vi "TeledyneMFC.vi"(7 "Value to Output":dbl format="%.2f", 8 "Ch Description":T1={"Ch Name"="TeleVue:Mdot:Meas(g/min)", "Type"="Run VI Named:", "Function"=enum."Analogue Output", "Ch State"=enum."On", "Calibration type"="Raw", "A"=0.0, "B"=0.0, "C"=0.0, "D"=0.0, "Comments"="!ASYNC", "Address"={"Main"=186, "Ch."=0, "Sub"=0, "Port Name"="tcp://192.168.124.71:10001"}, "String"="Front Panel", "Duty"=65535} {"Duty" format="%016b"; "D" format="%#_5g"; "C" format="%#_5g"; "B" format="%#_5g"; "A" format="%#_5g"}) -> (0 "Scan comment":string, 1 "Output":dbl=nan format="%.3f", 3 "HelpText":string="Analogue Input: Reads flowrate\nAnalogue Output: Sets digital control, sets setpoint, puts valve in auto\nNegative demand will ForceValveClosed\nDigital Output: 0-forceClosed, else-Automatic")   [LabVIEW 2017]
uses:
  ADAM Client/Sub VIs/ADAM Controls/Ch_description_ADAM.ctl
  ADAM Client/Sub VIs/ADAM Controls/Module_type_ADAM.ctl
  ADAM Client/Sub VIs/ADAM Controls/Function_ADAM.ctl
  ADAM Client/Sub VIs/ADAM Controls/Channel_State.ctl
  ADAM Client/Sub VIs/ADAM Controls/Calib_type_ADAM.ctl
  ADAM Client/Sub VIs/ADAM Controls/Address.ctl
  subVIs/TeledyneVueCommand.ctl
panel:
  out "GoodComms":bool
  # "VI to control Teledyne Vue Mass Flow Controller"
  # "http://www.teledyne-hi.com/products-services/thermal-mass-flow/300-vue-series"
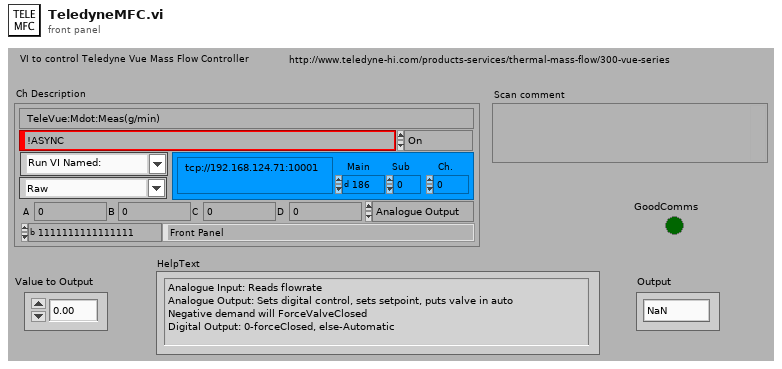
[diagram p1: front panel]
types:
  T1 = typedef "Ch_description_ADAM.ctl" = cluster{"Ch Name":string, "Type":T2, "Function":T3, "Ch State":T4, "Calibration type":T5, "A":dbl, "B":dbl, "C":dbl, "D":dbl, "Comments":string, "Address":T6, "String":string, "Duty":u16}
  T2 = typedef "Module_type_ADAM.ctl" = string
  T3 = typedef "Function_ADAM.ctl" = enum16{"Analogue Input", "Digital Input", "Event counter", "Event rate", "Analogue Output", "Digital Output", "Relay Output"}
  T4 = typedef "Channel_State.ctl" = enum16{"On", "Off", "Always On", "Always Off"}
  T5 = typedef "Calib_type_ADAM.ctl" = string
  T6 = typedef "Address.ctl" = cluster{"Main":i32, "Ch.":i32, "Sub":i32, "Port Name":string}
  T7 = typedef "TeledyneVueCommand.ctl" = string
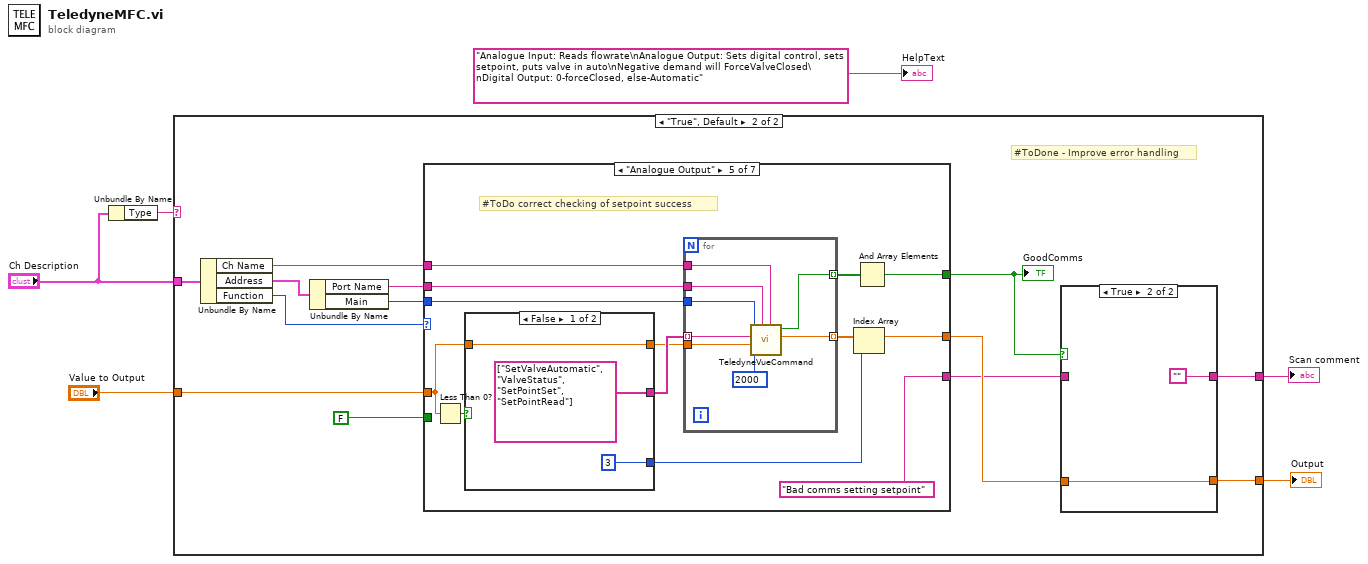
[diagram p0: block diagram]
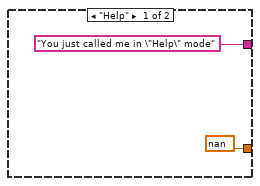
[diagram p2: hidden frame]
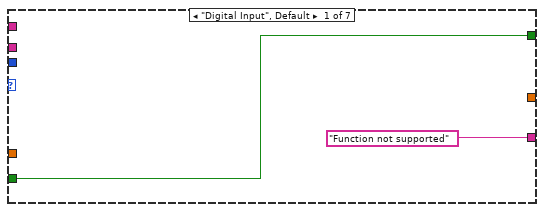
[diagram p3: hidden frame]
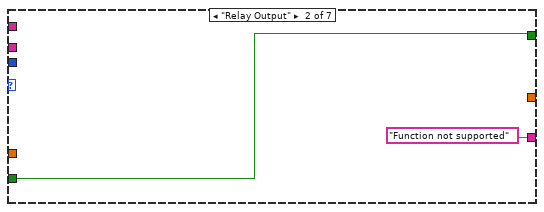
[diagram p4: hidden frame]
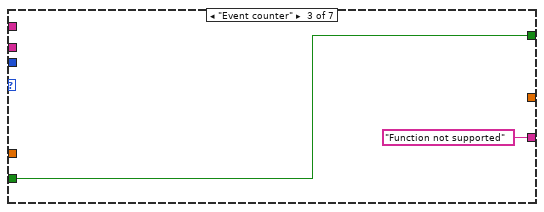
[diagram p5: hidden frame]
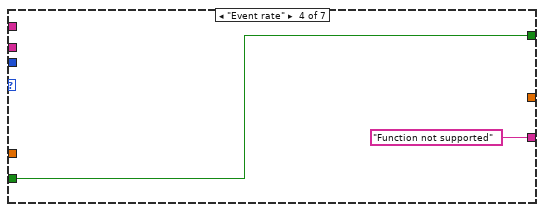
[diagram p6: hidden frame]
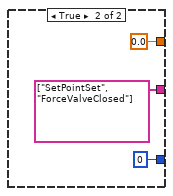
[diagram p7: hidden frame]
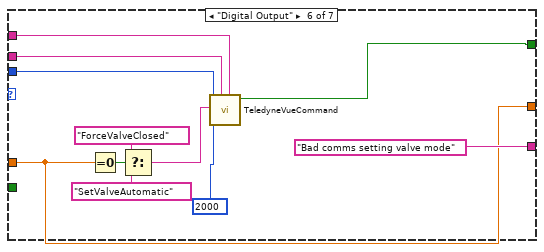
[diagram p8: hidden frame]
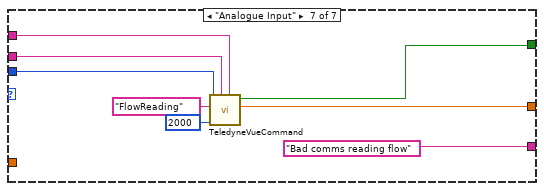
[diagram p9: hidden frame]
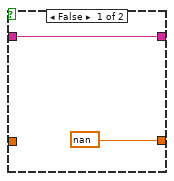
[diagram p10: hidden frame]
diagram:
  n1 = Unbundle By Name("Ch Description") -> ("Type"=w3:T2)
  n2 = case shown="\"True\", Default" w3 {
    tunnel: ["You just called me in \"Help\" mode" w20] -> w6
    tunnel: [nan ("t") w19] -> w5
    tunnel: "Ch Description" -> [_ w17]
    tunnel: "Value to Output" -> [_ w12]
    frame "Help" {
    }
    frame "True", Default {
      # "#ToDone - Improve error handling"
      n3 = Unbundle By Name(w17) -> ("Ch Name"=w13:string, "Address"=w21:T6, "Function"=w16:T3)
      n4 = Unbundle By Name(w21) -> ("Port Name"=w15:string, "Main"=w18:i32)
      n5 = case shown="\"Analogue Output\"" w16 {
        tunnel: w18 -> [_ _ _ _ w41 w66 w74]
        tunnel: w15 -> [_ _ _ _ w42 w67 w75]
        tunnel: [_ _ _ _ w37 w57 w72] -> w14
        tunnel: w13 -> [_ _ _ _ w40 w65 w71]
        tunnel: w12 -> [_ _ _ _ w32 w57 _]
        tunnel: [w23 w25 w27 w29 w35 w60 w70] -> w11
        tunnel: FALSE -> [w23 w25 w27 w29 _ _ _]
        tunnel: ["Function not supported" "Function not supported" "Function not supported" "Function not supported" "Bad comms setting setpoint" "Bad comms setting valve mode" "Bad comms reading flow"] -> w9
        frame "Digital Input", Default {
        }
        frame "Relay Output" {
        }
        frame "Event counter" {
        }
        frame "Event rate" {
        }
        frame "Analogue Output" {
          # "#ToDo correct checking of setpoint success"
          n6 = Less Than 0?(x=w32) -> (x < 0?=w33:bool)
          n7 = case shown="False" w33 {
            tunnel: [T7[] ["SetValveAutomatic", "ValveStatus", "SetPointSet", "SetPointRead"] T7[] ["SetPointSet", "ForceValveClosed"]] -> w38
            tunnel: w32 -> [w44 _]
            tunnel: [w44 0.0 ("Value to Output")] -> w31
            tunnel: [3 ("index") 0 ("index")] -> w30
            frame False {
            }
            frame True {
            }
          }
          n8 = for {
            tunnel: w42 -> [w56]
            tunnel: w41 -> [w55]
            tunnel: w38 -> [w54] mode=indexing
            tunnel: w40 -> [w53]
            tunnel: w31 -> [w51]
            tunnel: [w50] -> w39 mode=indexing
            tunnel: [w49] -> w36 mode=indexing
            n9 = call "TeledyneVueCommand.vi"("Channel Name"=w53, "Port Name"=w56, "Timeout/ms"=u32 2000, "Numeric Value"=w51, "TeledyneVueCommand"=w54, "Address"=w55) -> ("Numeric Reply"=w50:dbl, "OK"=w49:bool)  [unwired: 1 in, 2 out]
          }
          n10 = Index Array(array=w39, index=w30) -> (element=w37:dbl)
          n11 = And Array Elements(Boolean array=w36) -> (logical AND=w35:bool)
        }
        frame "Digital Output" {
          n12 = Equal To 0?(x=w57) -> (x = 0?=w64:bool)
          n13 = Select(t=T7 "ForceValveClosed" ("AalborgDFCCommand"), s=w64, f=T7 "SetValveAutomatic" ("AalborgDFCCommand")) -> (s? t:f=w61:T7)
          n14 = call "TeledyneVueCommand.vi"("Channel Name"=w65, "Port Name"=w67, "Timeout/ms"=u32 2000, "TeledyneVueCommand"=w61, "Address"=w66) -> ("OK"=w60:bool)  [unwired: 2 in, 3 out]
        }
        frame "Analogue Input" {
          n15 = call "TeledyneVueCommand.vi"("Channel Name"=w71, "Port Name"=w75, "Timeout/ms"=u32 2000, "TeledyneVueCommand"=T7 "FlowReading" ("AalborgDFCCommand"), "Address"=w74) -> ("Numeric Reply"=w72:dbl, "OK"=w70:bool)  [unwired: 2 in, 2 out]
        }
      }
      "GoodComms" <- w11
      n16 = case shown="True" w11 {
        tunnel: [w76 ""] -> w20
        tunnel: [nan ("t") w78] -> w19
        tunnel: w14 -> [_ w78]
        tunnel: w9 -> [w76 _]
        frame False {
        }
        frame True {
        }
      }
    }
  }
  "Output" <- w5
  "Scan comment" <- w6
  "HelpText" <- "Analogue Input: Reads flowrate\nAnalogue Output: Sets digital control, sets setpoint, puts valve in auto\nNegative demand will ForceValveClosed\nDigital Output: 0-forceClosed, else-Automatic"
